vi "Single SSC DCPower Configure Single Point Force DC Voltage Symmetric Limits.vi"(0 "DCPower SSC in":T1, 1 "Voltage Level Range (V)":dbl format="%#_6p", 2 "Current Limit Range (A)":dbl format="%#_6p", 5 "Voltage Level (V)":dbl format="%#_6p", 7 "Current Limit (A)":dbl format="%#_6p", 11 "error in":errorcluster) -> (4 "DCPower SSC out":T1, 15 "error out":errorcluster)   [LabVIEW 2020]
doc: "This VI configures the instrument sessions to force a single voltage."
uses:
  SSC DCPower.ctl
  <instrlib>/niDCPower/nidcpower.llb/niDCPower Source Mode.ctl
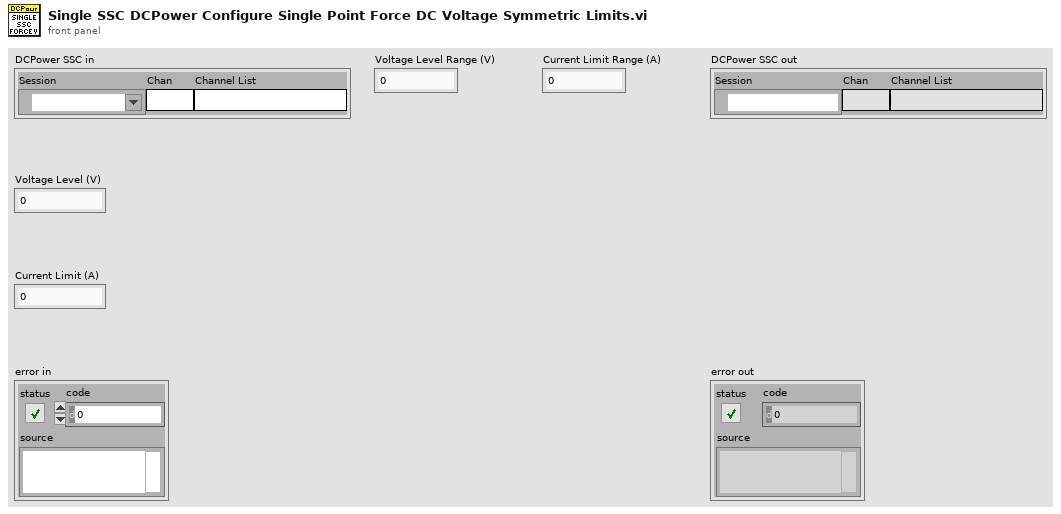
[diagram p1: front panel]
types:
  T1 = typedef "SSC DCPower.ctl" = cluster{"Session":refnum<k15>, "Chan":string, "Channel List":string}
  T2 = typedef "niDCPower Source Mode.ctl" = i32
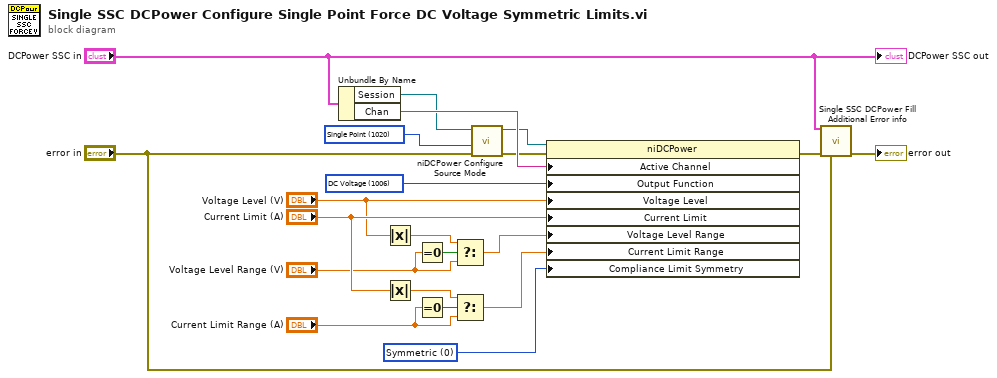
[diagram p0: block diagram]
diagram:
  w1 = 0 items=["Symmetric", "Asymmetric"] ("Source:Advanced:Compliance Limit Symmetry")
  w5 = T2 1020 items=["Single Point"=1020, "Sequence"=1021] ("source mode")
  w9 = 1006 items=["DC Voltage"=1006, "DC Current"=1007, "Pulse Voltage"=1049, "Pulse Current"=1050] ("Source:Output Function")
  n1 = Unbundle By Name("DCPower SSC in") -> ("Session"=w7:refnum<k15>, "Chan"=w10:string)
  n2 = Absolute Value(x="Voltage Level (V)") -> (abs(x)=w16:dbl)
  n3 = Absolute Value(x="Current Limit (A)") -> (abs(x)=w13:dbl)
  n4 = Equal To 0?(x="Voltage Level Range (V)") -> (x = 0?=w15:bool)
  n5 = Equal To 0?(x="Current Limit Range (A)") -> (x = 0?=w14:bool)
  n6 = Select(t=w16, s=w15, f="Voltage Level Range (V)") -> (s? t:f=w12:dbl)
  n7 = Select(t=w13, s=w14, f="Current Limit Range (A)") -> (s? t:f=w11:dbl)
  n8 = call <instrlib>:"niDCPower Configure Source Mode.vi"("error in (no error)"="error in", "source mode"=w5, "instrument handle"=w7) -> ("error out"=w8:errorcluster, "instrument handle out"=w6:refnum<k15>)  [unwired: 7 in]
  n9 = property class="niDCPower"(reference=w6, error in=w8, "Active Channel"=w10, "Output Function"=w9, "Voltage Level"="Voltage Level (V)", "Current Limit"="Current Limit (A)", "Voltage Level Range"=w12, "Current Limit Range"=w11, "Compliance Limit Symmetry"=w1) -> (error out=w20:errorcluster)  [unwired: 1 out]
  n10 = call "Single SSC DCPower Fill Additional Error info.vi"("DCPower SSC in"="DCPower SSC in", "error in"=w20, "previous error in"="error in") -> ("error out"=→"error out":errorcluster)  [unwired: 12 in]
  "DCPower SSC out" <- "DCPower SSC in"
